vi "Initialize.vi"(8 "error in":errorcluster, 11 "Plugin in":refnum<class "Output Sequencer.lvclass">) -> (0 "error out":errorcluster, 3 "Plugin out":refnum<class "Output Sequencer.lvclass">)   [LabVIEW 2024, in "Output Sequencer.lvlib" / "Output Sequencer.lvclass"]
uses:
  Output Sequencer.lvclass
  C:/Program Files/National Instruments/LabVIEW 2024/vi.lib/FlexLogger/SDK/PluginSDK.lvlibp/PEFClasses/SDK/Plugin/Plugin.lvclass
  <vilib>/FlexLogger/SDK/PluginSDK.lvlibp/PEFClasses/SDK/Processing Element/Timing Parameters.ctl
  <vilib>/FlexLogger/SDK/PluginSDK.lvlibp/PEFClasses/SDK/Processing Element/Timing Method.ctl
  Globals/Global Strings.vi
  <vilib>/FlexLogger/SDK/PluginSDK.lvlibp/PEFClasses/SDK/Plugin/ParameterAccess/Write Command.vi
  <vilib>/FlexLogger/SDK/PluginSDK.lvlibp/PEFClasses/SDK/Plugin/ParameterAccess/Write N Digital Channel.vi
  <vilib>/FlexLogger/SDK/PluginSDK.lvlibp/PEFClasses/SDK/Plugin/ParameterAccess/Write N Channel.vi
  <vilib>/FlexLogger/SDK/PluginSDK.lvlibp/PEFClasses/SDK/Plugin/Plugin.lvclass
  <vilib>/FlexLogger/SDK/PluginSDK.lvlibp/PEFClasses/SDK/Processing Element/Processing Element.lvclass
  C:/Program Files/National Instruments/LabVIEW 2024/vi.lib/FlexLogger/SDK/PluginSDK.lvlibp/PEFClasses/SDK/Processing Element/Processing Element.lvclass
  C:/Dev/GitHub/ni/niflexlogger-plugins/PDK plugins/Output Sequencer/source/Output Sequencer/Output Sequencer.lvclass
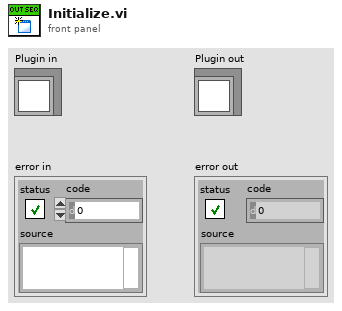
[diagram p1: front panel]
types:
  T1 = typedef "PluginSDK.lvlibp/Processing Element.lvclass/Timing Parameters.ctl" = cluster{"Timing Method":T2, "Timing Period (ms)":i32}
  T2 = typedef "PluginSDK.lvlibp/Processing Element.lvclass/Timing Method.ctl" = enum16{"Periodic", "Immediate", "On Data Ready", "Triggered"}
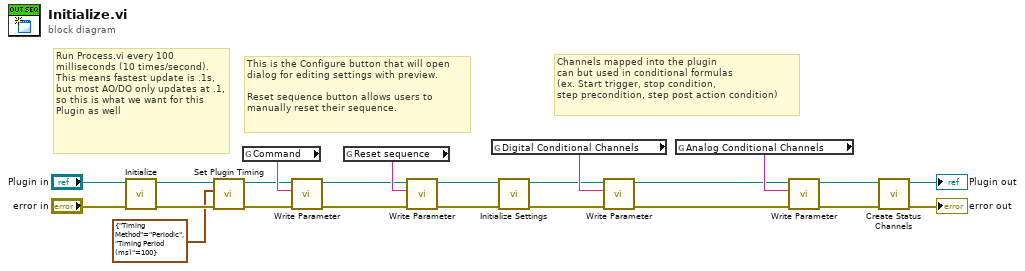
[diagram p0: block diagram]
diagram:
  # "Channels mapped into the plugin\ncan but used in conditional formulas\n(ex. Start trigger, stop condition,\nstep precondition, step post action condition)"
  # "This is the Configure button that will open\ndialog for editing settings with preview.\n\nReset sequence button allows users to\nmanually reset their sequence."
  # "Run Process.vi every 100 milliseconds (10 times/second). This means fastest update is .1s, but most AO/DO only updates at .1, so this is what we want for this Plugin as well"
  n1 = call-parent "Initialize.vi"("error in (no error)"="error in", "Plugin in"="Plugin in") -> ("error out"=w23:errorcluster, "Plugin out"=w21:refnum<class "Output Sequencer.lvclass">)  [unwired: 8 in]
  n2 = call <vilib>:"Set Plugin Timing.vi"("error in (no error)"=w23, "Timing Parameters"=T1 {"Timing Method"=enum."Periodic", "Timing Period (ms)"=100}, "Plugin in"=w21) -> ("error out"=w11:errorcluster, "Plugin out"=w12:refnum<class "Output Sequencer.lvclass">)  [unwired: 7 in]
  n3 = global read "Global Strings.vi" "Command"() -> (w20:string)
  n4 = call-poly <vilib>:"Write Parameter.vi"("error in (no error)"=w11, "Name"=w20, "Plugin in"=w12) -> ("error out"=w9:errorcluster, "Plugin out"=w10:refnum<class "Output Sequencer.lvclass">)  [unwired: 7 in]
  n5 = global read "Global Strings.vi" "Reset sequence"() -> (w13:string)
  n6 = call-poly <vilib>:"Write Parameter.vi"("error in (no error)"=w9, "Name"=w13, "Plugin in"=w10) -> ("error out"=w5:errorcluster, "Plugin out"=w4:refnum<class "Output Sequencer.lvclass">)  [unwired: 7 in]
  n7 = global read "Global Strings.vi" "Digital Conditional Channels"() -> (w19:string)
  n8 = call "Initialize Settings.vi"("error in (no error)"=w5, "Output Sequencer in"=w4) -> ("error out"=w2:errorcluster, "Output Sequencer out"=w3:refnum<class "Output Sequencer.lvclass">)  [unwired: 8 in]
  n9 = call-poly <vilib>:"Write Parameter.vi"("error in (no error)"=w2, "Name (Unique Channel Identifier)"=w19, "Plugin in"=w3) -> ("error out"=w17:errorcluster, "Plugin out"=w16:refnum<class "Output Sequencer.lvclass">)  [unwired: 7 in]
  n10 = global read "Global Strings.vi" "Analog Conditional Channels"() -> (w18:string)
  n11 = call-poly <vilib>:"Write Parameter.vi"("error in (no error)"=w17, "Name (Unique Channel Identifier)"=w18, "Plugin in"=w16) -> ("error out"=w8:errorcluster, "Plugin out"=w1:refnum<class "Output Sequencer.lvclass">)  [unwired: 7 in]
  n12 = call "Create Status Channels.vi"("error in (no error)"=w8, "Output Sequencer in"=w1) -> ("error out"=→"error out":errorcluster, "Output Sequencer out"=→"Plugin out":refnum<class "Output Sequencer.lvclass">)  [unwired: 8 in]
